vi "ProgG_004_MG.vi"() -> ()   [LabVIEW 2021]
panel:
  out "min(X,Y)":dbl=2.7183
  out "max(X,Y)":dbl=3.1416
  in  "Y":ext=2.7182999999999999999
  in  "X":ext=3.1416
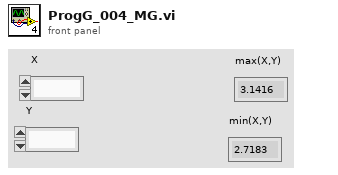
[diagram p1: front panel]
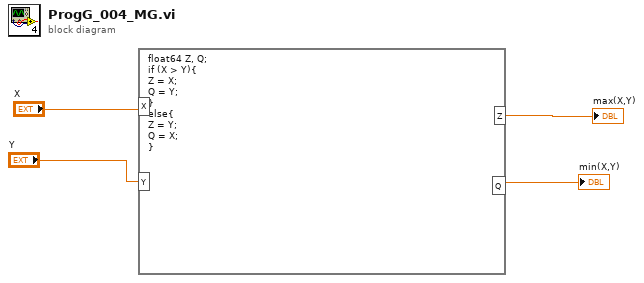
[diagram p0: block diagram]
diagram:
  n1 = formula code="float64 Z, Q;\nif (X > Y){\nZ = X;\nQ = Y;\n}\nelse{\nZ = Y;\nQ = X;\n}"("X"="X", "Y"="Y") -> ("Z"=→"max(X,Y)":dbl, "Q"=→"min(X,Y)":dbl)
